vi "Creat Font by Ref and Style.vi"(8 "error in (no error)":errorcluster caption="错误输入（无错误）", 10 "newStyle":i32(ring) items=["Regular"=0, "Bold"=1, "Italic"=2, "Underline"=4, "Strikeout"=8], 11 "prototype":refnum<k24>) -> (0 "error out":errorcluster caption="错误输出", 3 "new reference":refnum<k24>)   [LabVIEW 2011, in "Font.lvclass"]
uses:
  Font.lvclass
  System.Drawing
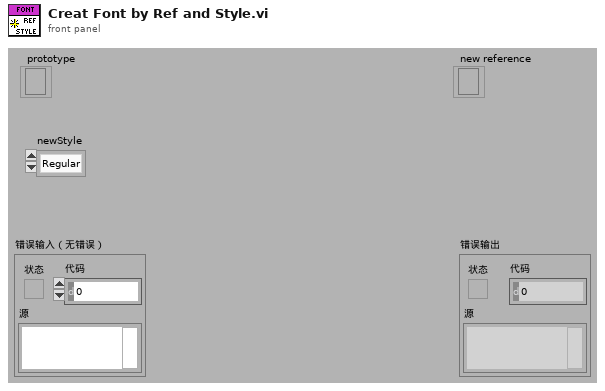
[diagram p1: front panel]
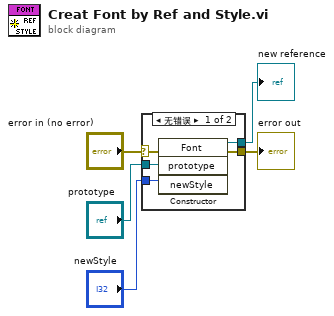
[diagram p0: block diagram]
diagram:
  n1 = case shown="无错误" "error in (no error)" {
    selector: "error in (no error)" -> [w10 w11]
    tunnel: [w7 w11] -> w4
    tunnel: "prototype" -> [w9 _]
    tunnel: "newStyle" -> [w8 _]
    tunnel: [w6 _] -> w1
    frame No Error {
      n2 = constructor class="Font"(error in=w10, "prototype"=w9, "newStyle"=w8) -> (reference out=w6:refnum<k24>, error out=w7:errorcluster)  [unwired: 2 in, 3 out]
    }
    frame Error {
    }
  }
  "error out" <- w4
  "new reference" <- w1
